vi "2dQuickSort(String).vi"(7 "Row?(F)":bool, 9 "Sort Index(0)":i32, 11 "Array In":string[][](array[string])) -> (2 "Out of Bounds?":bool, 3 "Array Out":string[][](array[string]))   [LabVIEW 2013, in "Sorting.lvlib"]
uses:
  Sorting.lvlib
  1d Sort With Indices/Quick Sort/SubVIs/QuickSort Instances/QuickSort(String).vi
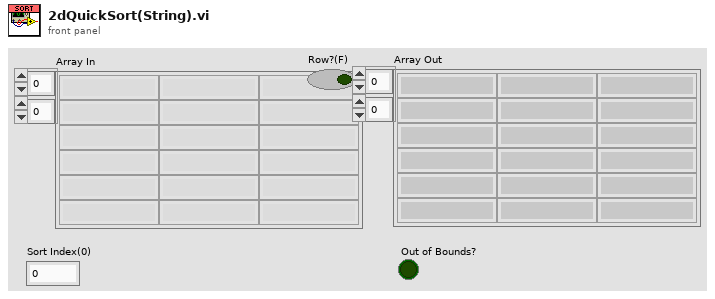
[diagram p1: front panel]
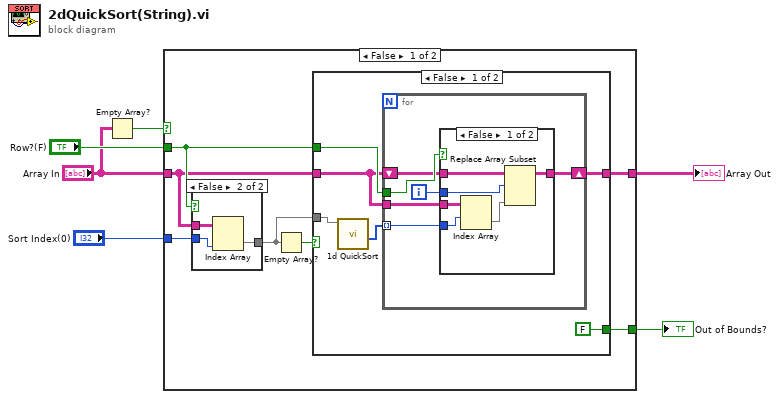
[diagram p0: block diagram]
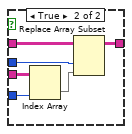
[diagram p2: hidden frame]
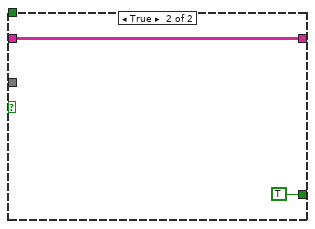
[diagram p3: hidden frame]
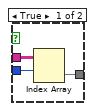
[diagram p4: hidden frame]
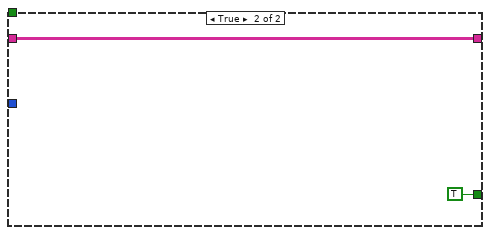
[diagram p5: hidden frame]
diagram:
  n1 = Empty Array?(array="Array In") -> (empty?=w2:bool)
  n2 = case shown="False" w2 {
    tunnel: "Sort Index(0)" -> [w13 _]
    tunnel: "Row?(F)" -> [w12 _]
    tunnel: [w11 w47] -> w4
    tunnel: "Array In" -> [w10 w47]
    tunnel: [w7 TRUE] -> w1
    frame False {
      n3 = case shown="False" w12 {
        tunnel: w10 -> [w42 w45]
        tunnel: [w41 w44] -> w9
        tunnel: w13 -> [w40 w43]
        frame True {
          n4 = Index Array(array=w42, index (row)=w40) -> (element=w41:string[])  [unwired: 1 in]
        }
        frame False {
          n5 = Index Array(array=w45, index (col)=w43) -> (element=w44:string[])  [unwired: 1 in]
        }
      }
      n6 = Empty Array?(array=w9) -> (empty?=w8:bool)
      n7 = case shown="False" w8 {
        tunnel: w12 -> [w19 _]
        tunnel: [w18 w39] -> w11
        tunnel: w10 -> [w17 w39]
        tunnel: w9 -> [w15 _]
        tunnel: [FALSE TRUE] -> w7
        frame False {
          n8 = call-poly "1d QuickSort.vi"("Array In"=w15) -> ("Indices Out"=w14:i32[])  [unwired: 9 in, 1 out]
          n9 = for {
            tunnel: w14 -> [w20] mode=indexing
            tunnel: w17 -> [w24]
            tunnel: w19 -> [w25]
            shift-right: [w22] -> w18
            shift-left: w17 -> [w23]
            i -> [w21]
            n10 = case shown="False" w25 {
              tunnel: w24 -> [w31 w37]
              tunnel: w20 -> [w27 w34]
              tunnel: w23 -> [w30 w36]
              tunnel: [w28 w33] -> w22
              tunnel: w21 -> [w26 w32]
              frame False {
                n11 = Index Array(array=w31, index (row)=w27) -> (element=w29:string[])  [unwired: 1 in]
                n12 = Replace Array Subset(array=w30, new element=w29, index (row)=w26) -> (w28:string[][])  [unwired: 1 in]
              }
              frame True {
                n13 = Index Array(array=w37, index (col)=w34) -> (element=w35:string[])  [unwired: 1 in]
                n14 = Replace Array Subset(array=w36, new element=w35, index (col)=w32) -> (w33:string[][])  [unwired: 1 in]
              }
            }
          }
        }
        frame True {
        }
      }
    }
    frame True {
    }
  }
  "Array Out" <- w4
  "Out of Bounds?" <- w1
